vi "correct_juese.vi"(6 "juese":string, 9 "fqren":string) -> (0 "error 2":errorcluster caption="error out 10", 2 "nx_juese":string)   [LabVIEW 2017, in "Lib_code.lvlib"]
uses:
  Lib_code.lvlib
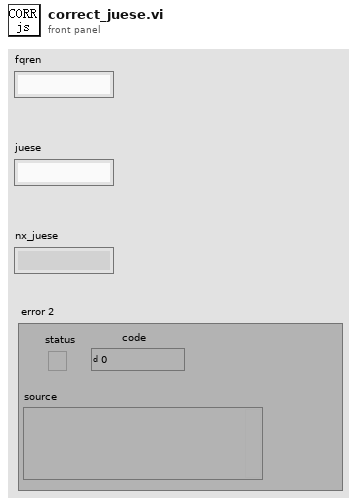
[diagram p1: front panel]
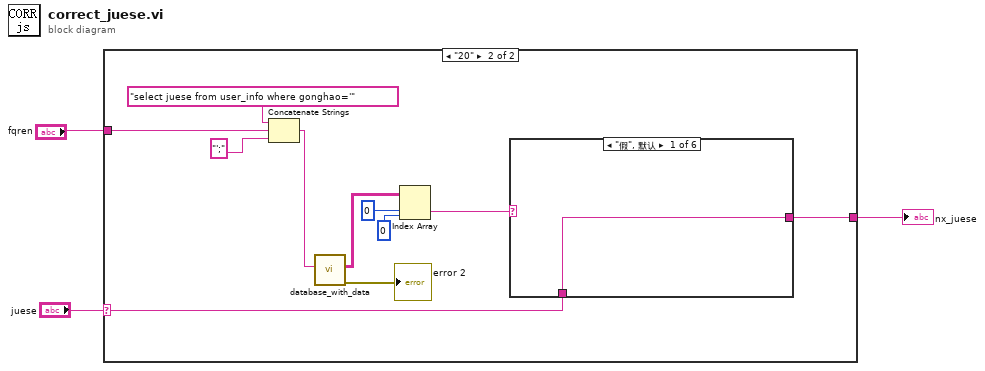
[diagram p0: block diagram]
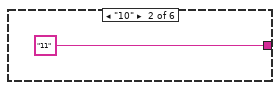
[diagram p3: hidden frame]
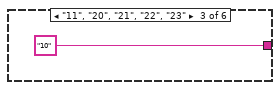
[diagram p4: hidden frame]
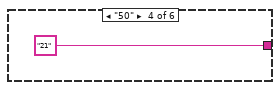
[diagram p5: hidden frame]
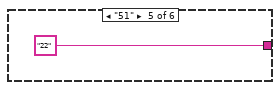
[diagram p6: hidden frame]
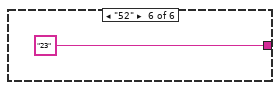
[diagram p7: hidden frame]
diagram:
  n1 = case shown="\"20\"" "juese" {
    selector: "juese" -> [w4 w5]
    tunnel: [w4 w7] -> w2
    tunnel: "fqren" -> [_ w11]
    frame "假", Default {
    }
    frame "20" {
      n2 = Concatenate Strings("select juese from user_info where gonghao='" ("Command Text"), w11, "';" ("字符串")) -> (w13:string)
      n3 = call "database_with_data.vi"("input"=w13) -> ("error"=→"error 2":errorcluster, "Data"=w8:string[][])  [unwired: 9 in]
      n4 = Index Array(array=w8, index (row)=0 ("索引 (行)"), index (col)=0 ("禁用的索引 (列)")) -> (element=w6:string)
      n5 = case shown="\"假\", 默认" w6 {
        tunnel: [w16 "11" ("y") "10" ("y") "21" ("y") "22" ("y") "23" ("y")] -> w7
        tunnel: w5 -> [w16 _ _ _ _ _]
        frame "假", Default {
        }
        frame "10" {
        }
        frame "11", "20", "21", "22", "23" {
        }
        frame "50" {
        }
        frame "51" {
        }
        frame "52" {
        }
      }
    }
  }
  "nx_juese" <- w2
